vi "Signal Driver.vi"() -> ()   [LabVIEW 2010]
doc: "This version of Signal Driver uses a different file access option for method files and thus it can not open method files created with the previous version.\n\n\nSignal Driver is a general purpose signal generator that was designed to control experiments that required repeatable timing over widely varied time scales. Signal Driver provides an easy framework for creating analog waveforms that cycle on an off while retaining exact synchronization. Complex sequences of warm up and cycling of control signals during an experiment can be easily created using the warm up and program controls. The need for this software was Particle Tracking Velocimetry and Laser Induced Fluorescence in a wave tank. Signal Driver was designed to control the wavemaker, lasers, rotating mirror, shutter, and high speed digital camera while providing precise control of the phase relationships. \n\nThe main screen of the Signal Driver has 4 controls and a boolean control palette.\n\nramp time (s) - The number of seconds during which time the Analog output signals ramp to the last value in their waveform arrays. The ramping occurs using a sinusoidal curve. The ramping is designed to prevent damage to any devices that would suffer from a large instantaneous change in control voltage. Note that the ramp is to the LAST value, not to the first value in the waveform arrays. The assumption is that the waveforms are continuous and cyclic.\n\nWarm up - An array containg boolean switches for each of the channels as well as the number of times each element in the array is to be repeated.\n\nThe warm up control is the first part of the program and the array must contain at least one element. For each element in the warm up array Signal Driver writes one repeat period of signal to each channel n times based on the status of the boolean controls. Additional elements can be added by using the index control and then setting the boolean switches and n to the desired values. Channels that are turned off receive a constant analog voltage equal to the last voltage in their waveform array.\n\nRight click on the index to empty the array.\n\nProgram\nThe Program control is identical to the warm up control. The only difference is that the program cycles the number of times indicated by the program cycles control.\n\nProgram Cycles\nNumber of times that the program array is cycled through.\n\nControl Palette\nContains controls for setting waveforms, ramping to the start position, sending the programmed signals, ramping to zero, and quitting. The controls are dimmed when they are disabled."
uses:
  AO Write (waveform).vi
  AO Write (scaled array).vi
  wavecluster.ctl
  AO n wave.ctl
  SDMethod.ctl
panel:
  in  "Del warmup":bool
  in  "Del program":bool
  out "period (s)":dbl=2.0 format="%.2f"
  out "actual update rate":sgl=1000.0 format="%.8f"
  out "SD method":T1 {"method array"."offset" format="%.2f"; "method array"."amplitude" format="%.2f"; "method array"."cycles/repeat period" min=1}
  out "last value":dbl[](array[numeric])=[-6.999965667724609] format="%.2f"
  in  "program":T2[](array[typedef])=[{"n"=1, "on/off"=[TRUE, FALSE, FALSE, FALSE, FALSE, FALSE]}] {"n" min=1}
  out "ready to run":cluster{"ramped":bool, "got waveforms":bool}={"ramped"=FALSE, "got waveforms"=TRUE}
  out "delay":i32=500
  out "end of cycle":i32=1002
  out "program cycles done":i32(slide)=1 scale=0.0..1.0
  out "wave periods":i32=107
  in  "program cycles":i32=1 min=1
  in  "warm up":T2[](array[typedef])=[{"n"=1, "on/off"=[FALSE, FALSE, FALSE, FALSE, FALSE, FALSE]}] {"n" min=1}
  in  "buffer size":i32=2000
  in  "State":T3
  in  "ramp time (s)":dbl=2.0 min=1.0 step=0.1 format="%.1f"
  in  "ramp points":i32=1000 min=100 max=10000
  out "waveform array":T4=[[-7.0, -6.9999657, -6.9998617, -6.999689, -6.9994473, -6.9991364, -6.9987564, -6.998307, -6.9977894, -6.997202, -6.996546, -6.9958205, -6.995026, -6.994163, -6.9932303, -6.992229, -6.9911585, -6.9900193, -6.988811, -6.9875336, -6.986187, -6.9847717, -6.9832873, -6.9817343, -6.980112, -6.978421, -6.9766617, -6.974833, -6.972935, -6.9709687, -6.9689336, -6.96683, -6.9646573, -6.9624157, -6.9601054, -6.9577265, -6.9552794, -6.952763, -6.950178, -6.947525, -6.9448028, -6.9420123, -6.939153, -6.936226, -6.93323, -6.930166, -6.927033, -6.9238315, -6.9205623, -6.9172244, -6.9138184, -6.910344, -6.9068017, -6.903191, -6.8995123, -6.8957653, -6.89195, -6.8880672, -6.8841166, -6.8800974, -6.876011, -6.871856, -6.867634, -6.8633432, -6.8589854, -6.85456, -6.850066, -6.845505, -6.840877, -6.8361807, -6.8314176, -6.8265862, -6.821688, -6.8167224, -6.8116894, -6.8065896, -6.801422, -6.796188, -6.7908864, -6.7855177, -6.780082, -6.7745795, -6.7690105, -6.7633743, -6.7576714, -6.751902, -6.7460656, -6.740163, -6.734194, -6.728158, -6.722056, -6.715887, -6.7096524, -6.7033515, -6.6969843, -6.6905513, -6.684052, -6.6774864, -6.6708555, -6.6641583, -6.657396, -6.650567, -6.643673, -6.6367135, -6.6296883, -6.6225977, -6.6154413, -6.60822, -6.6009336, -6.593582, -6.5861654, -6.578684, -6.571137, -6.5635257, -6.555849, -6.548108, -6.5403028, -6.5324326, -6.524498, -6.5164986, -6.5084352, -6.500308, -6.492116, -6.4838605, -6.4755406, -6.467157, -6.4587092, -6.4501977, -6.4416227, -6.4329844, -6.4242826, -6.415517, -6.406688, -6.397796, -6.388841, -6.3798227, -6.370742, -6.361598, -6.352391, -6.3431215, -6.3337893, -6.3243947, -6.3149376, -6.3054185, -6.295837, -6.286193, -6.2764874, -6.2667193, -6.25689, -6.246999, -6.237046, -6.227031, -6.216955, -6.2068176, -6.196619, -6.1863594, -6.1760387, -6.1656566, -6.1552143, -6.144711, -6.1341467, -6.1235223, -6.1128373, -6.102092, -6.091286, -6.0804205, -6.0694947, -6.0585093, -6.047464, -6.036359, -6.025194, -6.01397, -6.0026865, -5.991344, -5.979942, -5.968481, -5.956961, -5.9453826, -5.9337454, -5.9220495, -5.9102955, -5.898483, -5.886612, -5.8746834, -5.862696, -5.8506517, -5.838549, -5.826389, -5.8141713, -5.801896, -5.789564, -5.7771745, -5.764728, -5.752225, -5.7396646, -5.727048, -5.7143745, -5.701645, -5.688859, -5.6760173, -5.663119, -5.650165, -5.637155, -5.6240897, -5.610969, -5.5977926, -5.584561, -5.5712743, -5.557933, -5.544536, -5.531085, -5.517579, -5.5040193, -5.4904046, -5.4767356, -5.4630127, -5.449236, -5.4354057, -5.421521, -5.4075837, -5.393593, -5.3795485, -5.365451, -5.3513007, -5.3370976, -5.3228416, -5.308533, -5.294173, -5.27976, -5.2652946, -5.2507777, -5.2362084, -5.221588, -5.206916, -5.1921926, -5.1774178, -5.162592, -5.147715, -5.132787, -5.1178093, -5.1027803, -5.0877013, -5.0725718, -5.0573926, -5.0421634, -5.026884, -5.011555, -4.996177, -4.9807496, -4.965273, -4.9497476, -4.934173, -4.91855, -4.9028783, -4.887158, -4.8713894, -4.855573, -4.839709, -4.8237967, -4.807837, -4.7918296, -4.7757754, -4.7596736, -4.743525, -4.7273297, -4.7110877, -4.694799, -4.678464, -4.662083, -4.645656, -4.6291833, -4.612664, -4.5961003, -4.5794907, -4.562836, -4.5461364, -4.529392, -4.5126023, -4.4957685, -4.4788904, -4.461968, -4.4450016, -4.427991, -4.4109373, -4.3938394, -4.3766985, -4.359514, -4.3422875, -4.3250175, -4.3077044, -4.2903495, -4.2729516, -4.255512, -4.2380304, -4.2205067, -4.2029414, -4.1853347, -4.167687, -4.1499977, -4.1322675, -4.1144967, -4.0966854, -4.0788336, -4.060941, -4.043009, -4.025037, -4.007025, -3.9889734, -3.9708827, -3.9527526, -3.9345837, -3.9163759, -3.8981292, -3.8798444, -3.861521, -3.8431597, -3.8247604, -3.8063233, -3.7878487, -3.7693367, -3.7507875, -3.7322013, -3.7135782, -3.6949186, -3.6762223, -3.65749, -3.6387215, -3.619917, -3.6010768, -3.582201, -3.5632899, -3.5443437, -3.5253625, -3.5063465, -3.4872956, -3.4682107, -3.4490914, -3.429938, -3.4107509, -3.39153, -3.3722758, -3.352988, -3.3336675, -3.314314, -3.2949276, -3.2755086, -3.2560575, -3.2365742, -3.2170591, -3.1975121, -3.1779335, -3.1583235, -3.1386826, -3.1190104, -3.0993075, -3.079574, -3.0598104, -3.0400164, -3.0201924, -3.0003386, -2.9804552, -2.9605422, -2.9406002, -2.920629, -2.900629, -2.8806005, -2.8605435, -2.8404584, -2.8203452, -2.800204, -2.7800353, -2.759839, -2.7396157, -2.7193651, -2.6990879, -2.6787841, -2.6584537, -2.638097, -2.6177144, -2.597306, -2.5768719, -2.5564122, -2.5359275, -2.5154178, -2.494883, -2.474324, -2.4537404, -2.4331324, -2.4125004, -2.3918447, -2.3711655, -2.3504627, -2.3297367, -2.3089879, -2.288216, -2.267422, -2.2466052, -2.2257664, -2.2049057, -2.1840231, -2.163119, -2.1421936, -2.1212468, -2.1002793, -2.079291, -2.0582824, -2.0372531, -2.0162039, -1.9951348, -1.974046, -1.9529377, -1.9318101, -1.9106636, -1.8894981, -1.8683139, -1.8471113, -1.8258905, -1.8046517, -1.783395, -1.7621208, -1.7408292, -1.7195204, -1.6981946, -1.6768521, -1.655493, -1.6341176, -1.612726, -1.5913185, -1.5698953, -1.5484567, -1.5270027, -1.5055337, -1.4840498, -1.4625512, -1.4410383, -1.4195111, -1.3979698, -1.3764149, -1.3548462, -1.3332644, -1.3116692, -1.2900611, -1.2684404, -1.246807, -1.2251614, -1.2035037, -1.1818341, -1.1601529, -1.1384602, -1.1167562, -1.0950413, -1.0733155, -1.0515791, -1.0298324, -1.0080755, -0.98630863, -0.964532, -0.9427459, -0.92095053, -0.899146, -0.8773326, -0.8555106, -0.8336801, -0.8118414, -0.7899947, -0.7681402, -0.7462781, -0.7244086, -0.702532, -0.68064845, -0.65875816, -0.63686144, -0.6149584, -0.5930492, -0.57113427, -0.54921365, -0.52728766, -0.50535643, -0.4834202, -0.4614792, -0.43953365, -0.41758376, -0.39562973, -0.37367183, -0.35171023, -0.32974514, -0.30777684, -0.28580546, -0.2638313, -0.24185449, -0.21987532, -0.19789396, -0.17591067, -0.15392563, -0.13193908, -0.10995122, -0.08796228, -0.06597247, -0.043982007, -0.021991113, 1.08586066e-13, 0.021991113, 0.043982007, 0.06597247, 0.08796228, 0.10995122, 0.13193908, 0.15392563, 0.17591067, 0.19789396, 0.21987532, 0.24185449, 0.2638313, 0.28580546, 0.30777684, 0.32974514, 0.35171023, 0.37367183, 0.39562973, 0.41758376, 0.43953365, 0.4614792, 0.4834202, 0.50535643, 0.52728766, 0.54921365, 0.57113427, 0.5930492, 0.6149584, 0.63686144, 0.65875816, 0.68064845, 0.702532, 0.7244086, 0.7462781, 0.7681402, 0.7899947, 0.8118414, 0.8336801, 0.8555106, 0.8773326, 0.899146, 0.92095053, 0.9427459, 0.964532, 0.98630863, 1.0080755, 1.0298324, 1.0515791, 1.0733155, 1.0950413, 1.1167562, 1.1384602, 1.1601529, 1.1818341, 1.2035037, 1.2251614, 1.246807, 1.2684404, 1.2900611, 1.3116692, 1.3332644, 1.3548462, 1.3764149, 1.3979698, 1.4195111, 1.4410383, 1.4625512, 1.4840498, 1.5055337, 1.5270027, 1.5484567, 1.5698953, 1.5913185, 1.612726, 1.6341176, 1.655493, 1.6768521, 1.6981946, 1.7195204, 1.7408292, 1.7621208, 1.783395, 1.8046517, 1.8258905, 1.8471113, 1.8683139, 1.8894981, 1.9106636, 1.9318101, 1.9529377, 1.974046, 1.9951348, 2.0162039, 2.0372531, 2.0582824, 2.079291, 2.1002793, 2.1212468, 2.1421936, 2.163119, 2.1840231, 2.2049057, 2.2257664, 2.2466052, 2.267422, 2.288216, 2.3089879, 2.3297367, 2.3504627, 2.3711655, 2.3918447, 2.4125004, 2.4331324, 2.4537404, 2.474324, 2.494883, 2.5154178, 2.5359275, 2.5564122, 2.5768719, 2.597306, 2.6177144, 2.638097, 2.6584537, 2.6787841, 2.6990879, 2.7193651, 2.7396157, 2.759839, 2.7800353, 2.800204, 2.8203452, 2.8404584, 2.8605435, 2.8806005, 2.900629, 2.920629, 2.9406002, 2.9605422, 2.9804552, 3.0003386, 3.0201924, 3.0400164, 3.0598104, 3.079574, 3.0993075, 3.1190104, 3.1386826, 3.1583235, 3.1779335, 3.1975121, 3.2170591, 3.2365742, 3.2560575, 3.2755086, 3.2949276, 3.314314, 3.3336675, 3.352988, 3.3722758, 3.39153, 3.4107509, 3.429938, 3.4490914, 3.4682107, 3.4872956, 3.5063465, 3.5253625, 3.5443437, 3.5632899, 3.582201, 3.6010768, 3.619917, 3.6387215, 3.65749, 3.6762223, 3.6949186, 3.7135782, 3.7322013, 3.7507875, 3.7693367, 3.7878487, 3.8063233, 3.8247604, 3.8431597, 3.861521, 3.8798444, 3.8981292, 3.9163759, 3.9345837, 3.9527526, 3.9708827, 3.9889734, 4.007025, 4.025037, 4.043009, 4.060941, 4.0788336, 4.0966854, 4.1144967, 4.1322675, 4.1499977, 4.167687, 4.1853347, 4.2029414, 4.2205067, 4.2380304, 4.255512, 4.2729516, 4.2903495, 4.3077044, 4.3250175, 4.3422875, 4.359514, 4.3766985, 4.3938394, 4.4109373, 4.427991, 4.4450016, 4.461968, 4.4788904, 4.4957685, 4.5126023, 4.529392, 4.5461364, 4.562836, 4.5794907, 4.5961003, 4.612664, 4.6291833, 4.645656, 4.662083, 4.678464, 4.694799, 4.7110877, 4.7273297, 4.743525, 4.7596736, 4.7757754, 4.7918296, 4.807837, 4.8237967, 4.839709, 4.855573, 4.8713894, 4.887158, 4.9028783, 4.91855, 4.934173, 4.9497476, 4.965273, 4.9807496, 4.996177, 5.011555, 5.026884, 5.0421634, 5.0573926, 5.0725718, 5.0877013, 5.1027803, 5.1178093, 5.132787, 5.147715, 5.162592, 5.1774178, 5.1921926, 5.206916, 5.221588, 5.2362084, 5.2507777, 5.2652946, 5.27976, 5.294173, 5.308533, 5.3228416, 5.3370976, 5.3513007, 5.365451, 5.3795485, 5.393593, 5.4075837, 5.421521, 5.4354057, 5.449236, 5.4630127, 5.4767356, 5.4904046, 5.5040193, 5.517579, 5.531085, 5.544536, 5.557933, 5.5712743, 5.584561, 5.5977926, 5.610969, 5.6240897, 5.637155, 5.650165, 5.663119, 5.6760173, 5.688859, 5.701645, 5.7143745, 5.727048, 5.7396646, 5.752225, 5.764728, 5.7771745, 5.789564, 5.801896, 5.8141713, 5.826389, 5.838549, 5.8506517, 5.862696, 5.8746834, 5.886612, 5.898483, 5.9102955, 5.9220495, 5.9337454, 5.9453826, 5.956961, 5.968481, 5.979942, 5.991344, 6.0026865, 6.01397, 6.025194, 6.036359, 6.047464, 6.0585093, 6.0694947, 6.0804205, 6.091286, 6.102092, 6.1128373, 6.1235223, 6.1341467, 6.144711, 6.1552143, 6.1656566, 6.1760387, 6.1863594, 6.196619, 6.2068176, 6.216955, 6.227031, 6.237046, 6.246999, 6.25689, 6.2667193, 6.2764874, 6.286193, 6.295837, 6.3054185, 6.3149376, 6.3243947, 6.3337893, 6.3431215, 6.352391, 6.361598, 6.370742, 6.3798227, 6.388841, 6.397796, 6.406688, 6.415517, 6.4242826, 6.4329844, 6.4416227, 6.4501977, 6.4587092, 6.467157, 6.4755406, 6.4838605, 6.492116, 6.500308, 6.5084352, 6.5164986, 6.524498, 6.5324326, 6.5403028, 6.548108, 6.555849, 6.5635257, 6.571137, 6.578684, 6.5861654, 6.593582, 6.6009336, 6.60822, 6.6154413, 6.6225977, 6.6296883, 6.6367135, 6.643673, 6.650567, 6.657396, 6.6641583, 6.6708555, 6.6774864, 6.684052, 6.6905513, 6.6969843, 6.7033515, 6.7096524, 6.715887, 6.722056, 6.728158, 6.734194, 6.740163, 6.7460656, 6.751902, 6.7576714, 6.7633743, 6.7690105, 6.7745795, 6.780082, 6.7855177, 6.7908864, 6.796188, 6.801422, 6.8065896, 6.8116894, 6.8167224, 6.821688, 6.8265862, 6.8314176, 6.8361807, 6.840877, 6.845505, 6.850066, 6.85456, 6.8589854, 6.8633432, 6.867634, 6.871856, 6.876011, 6.8800974, 6.8841166, 6.8880672, 6.89195, 6.8957653, 6.8995123, 6.903191, 6.9068017, 6.910344, 6.9138184, 6.9172244, 6.9205623, 6.9238315, 6.927033, 6.930166, 6.93323, 6.936226, 6.939153, 6.9420123, 6.9448028, 6.947525, 6.950178, 6.952763, 6.9552794, 6.9577265, 6.9601054, 6.9624157, 6.9646573, 6.96683, 6.9689336, 6.9709687, 6.972935, 6.974833, 6.9766617, 6.978421, 6.980112, 6.9817343, 6.9832873, 6.9847717, 6.986187, 6.9875336, 6.988811, 6.9900193, 6.9911585, 6.992229, 6.9932303, 6.994163, 6.995026, 6.9958205, 6.996546, 6.997202, 6.9977894, 6.998307, 6.9987564, 6.9991364, 6.9994473, 6.999689, 6.9998617, 6.9999657, 7.0, 6.9999657, 6.9998617, 6.999689, 6.9994473, 6.9991364, 6.9987564, 6.998307, 6.9977894, 6.997202, 6.996546, 6.9958205, 6.995026, 6.994163, 6.9932303, 6.992229, 6.9911585, 6.9900193, 6.988811, 6.9875336, 6.986187, 6.9847717, 6.9832873, 6.9817343, 6.980112, 6.978421, 6.9766617, 6.974833, 6.972935, 6.9709687, 6.9689336, 6.96683, 6.9646573, 6.9624157, 6.9601054, 6.9577265, 6.9552794, 6.952763, 6.950178, 6.947525, 6.9448028, 6.9420123, 6.939153, 6.936226, 6.93323, 6.930166, 6.927033, 6.9238315, 6.9205623, 6.9172244, 6.9138184, 6.910344, 6.9068017, 6.903191, 6.8995123, 6.8957653, 6.89195, 6.8880672, 6.8841166, 6.8800974, 6.876011, 6.871856, 6.867634, 6.8633432, 6.8589854, 6.85456, 6.850066, 6.845505, 6.840877, 6.8361807, 6.8314176, 6.8265862, 6.821688, 6.8167224, 6.8116894, 6.8065896, 6.801422, 6.796188, 6.7908864, 6.7855177, 6.780082, 6.7745795, 6.7690105, 6.7633743, 6.7576714, 6.751902, 6.7460656, 6.740163, 6.734194, 6.728158, 6.722056, 6.715887, 6.7096524, 6.7033515, 6.6969843, 6.6905513, 6.684052, 6.6774864, 6.6708555, 6.6641583, 6.657396, 6.650567, 6.643673, 6.6367135, 6.6296883, 6.6225977, 6.6154413, 6.60822, 6.6009336, 6.593582, 6.5861654, 6.578684, 6.571137, 6.5635257, 6.555849, 6.548108, 6.5403028, 6.5324326, 6.524498, 6.5164986, 6.5084352, 6.500308, 6.492116, 6.4838605, 6.4755406, 6.467157, 6.4587092, 6.4501977, 6.4416227, 6.4329844, 6.4242826, 6.415517, 6.406688, 6.397796, 6.388841, 6.3798227, 6.370742, 6.361598, 6.352391, 6.3431215, 6.3337893, 6.3243947, 6.3149376, 6.3054185, 6.295837, 6.286193, 6.2764874, 6.2667193, 6.25689, 6.246999, 6.237046, 6.227031, 6.216955, 6.2068176, 6.196619, 6.1863594, 6.1760387, 6.1656566, 6.1552143, 6.144711, 6.1341467, 6.1235223, 6.1128373, 6.102092, 6.091286, 6.0804205, 6.0694947, 6.0585093, 6.047464, 6.036359, 6.025194, 6.01397, 6.0026865, 5.991344, 5.979942, 5.968481, 5.956961, 5.9453826, 5.9337454, 5.9220495, 5.9102955, 5.898483, 5.886612, 5.8746834, 5.862696, 5.8506517, 5.838549, 5.826389, 5.8141713, 5.801896, 5.789564, 5.7771745, 5.764728, 5.752225, 5.7396646, 5.727048, 5.7143745, 5.701645, 5.688859, 5.6760173, 5.663119, 5.650165, 5.637155, 5.6240897, 5.610969, 5.5977926, 5.584561, 5.5712743, 5.557933, 5.544536, 5.531085, 5.517579, 5.5040193, 5.4904046, 5.4767356, 5.4630127, 5.449236, 5.4354057, 5.421521, 5.4075837, 5.393593, 5.3795485, 5.365451, 5.3513007, 5.3370976, 5.3228416, 5.308533, 5.294173, 5.27976, 5.2652946, 5.2507777, 5.2362084, 5.221588, 5.206916, 5.1921926, 5.1774178, 5.162592, 5.147715, 5.132787, 5.1178093, 5.1027803, 5.0877013, 5.0725718, 5.0573926, 5.0421634, 5.026884, 5.011555, 4.996177, 4.9807496, 4.965273, 4.9497476, 4.934173, 4.91855, 4.9028783, 4.887158, 4.8713894, 4.855573, 4.839709, 4.8237967, 4.807837, 4.7918296, 4.7757754, 4.7596736, 4.743525, 4.7273297, 4.7110877, 4.694799, 4.678464, 4.662083, 4.645656, 4.6291833, 4.612664, 4.5961003, 4.5794907, 4.562836, 4.5461364, 4.529392, 4.5126023, 4.4957685, 4.4788904, 4.461968, 4.4450016, 4.427991, 4.4109373, 4.3938394, 4.3766985, 4.359514, 4.3422875, 4.3250175, 4.3077044, 4.2903495, 4.2729516, 4.255512, 4.2380304, 4.2205067, 4.2029414, 4.1853347, 4.167687, 4.1499977, 4.1322675, 4.1144967, 4.0966854, 4.0788336, 4.060941, 4.043009, 4.025037, 4.007025, 3.9889734, 3.9708827, 3.9527526, 3.9345837, 3.9163759, 3.8981292, 3.8798444, 3.861521, 3.8431597, 3.8247604, 3.8063233, 3.7878487, 3.7693367, 3.7507875, 3.7322013, 3.7135782, 3.6949186, 3.6762223, 3.65749, 3.6387215, 3.619917, 3.6010768, 3.582201, 3.5632899, 3.5443437, 3.5253625, 3.5063465, 3.4872956, 3.4682107, 3.4490914, 3.429938, 3.4107509, 3.39153, 3.3722758, 3.352988, 3.3336675, 3.314314, 3.2949276, 3.2755086, 3.2560575, 3.2365742, 3.2170591, 3.1975121, 3.1779335, 3.1583235, 3.1386826, 3.1190104, 3.0993075, 3.079574, 3.0598104, 3.0400164, 3.0201924, 3.0003386, 2.9804552, 2.9605422, 2.9406002, 2.920629, 2.900629, 2.8806005, 2.8605435, 2.8404584, 2.8203452, 2.800204, 2.7800353, 2.759839, 2.7396157, 2.7193651, 2.6990879, 2.6787841, 2.6584537, 2.638097, 2.6177144, 2.597306, 2.5768719, 2.5564122, 2.5359275, 2.5154178, 2.494883, 2.474324, 2.4537404, 2.4331324, 2.4125004, 2.3918447, 2.3711655, 2.3504627, 2.3297367, 2.3089879, 2.288216, 2.267422, 2.2466052, 2.2257664, 2.2049057, 2.1840231, 2.163119, 2.1421936, 2.1212468, 2.1002793, 2.079291, 2.0582824, 2.0372531, 2.0162039, 1.9951348, 1.974046, 1.9529377, 1.9318101, 1.9106636, 1.8894981, 1.8683139, 1.8471113, 1.8258905, 1.8046517, 1.783395, 1.7621208, 1.7408292, 1.7195204, 1.6981946, 1.6768521, 1.655493, 1.6341176, 1.612726, 1.5913185, 1.5698953, 1.5484567, 1.5270027, 1.5055337, 1.4840498, 1.4625512, 1.4410383, 1.4195111, 1.3979698, 1.3764149, 1.3548462, 1.3332644, 1.3116692, 1.2900611, 1.2684404, 1.246807, 1.2251614, 1.2035037, 1.1818341, 1.1601529, 1.1384602, 1.1167562, 1.0950413, 1.0733155, 1.0515791, 1.0298324, 1.0080755, 0.98630863, 0.964532, 0.9427459, 0.92095053, 0.899146, 0.8773326, 0.8555106, 0.8336801, 0.8118414, 0.7899947, 0.7681402, 0.7462781, 0.7244086, 0.702532, 0.68064845, 0.65875816, 0.63686144, 0.6149584, 0.5930492, 0.57113427, 0.54921365, 0.52728766, 0.50535643, 0.4834202, 0.4614792, 0.43953365, 0.41758376, 0.39562973, 0.37367183, 0.35171023, 0.32974514, 0.30777684, 0.28580546, 0.2638313, 0.24185449, 0.21987532, 0.19789396, 0.17591067, 0.15392563, 0.13193908, 0.10995122, 0.08796228, 0.06597247, 0.043982007, 0.021991113, -6.395194e-13, -0.021991113, -0.043982007, -0.06597247, -0.08796228, -0.10995122, -0.13193908, -0.15392563, -0.17591067, -0.19789396, -0.21987532, -0.24185449, -0.2638313, -0.28580546, -0.30777684, -0.32974514, -0.35171023, -0.37367183, -0.39562973, -0.41758376, -0.43953365, -0.4614792, -0.4834202, -0.50535643, -0.52728766, -0.54921365, -0.57113427, -0.5930492, -0.6149584, -0.63686144, -0.65875816, -0.68064845, -0.702532, -0.7244086, -0.7462781, -0.7681402, -0.7899947, -0.8118414, -0.8336801, -0.8555106, -0.8773326, -0.899146, -0.92095053, -0.9427459, -0.964532, -0.98630863, -1.0080755, -1.0298324, -1.0515791, -1.0733155, -1.0950413, -1.1167562, -1.1384602, -1.1601529, -1.1818341, -1.2035037, -1.2251614, -1.246807, -1.2684404, -1.2900611, -1.3116692, -1.3332644, -1.3548462, -1.3764149, -1.3979698, -1.4195111, -1.4410383, -1.4625512, -1.4840498, -1.5055337, -1.5270027, -1.5484567, -1.5698953, -1.5913185, -1.612726, -1.6341176, -1.655493, -1.6768521, -1.6981946, -1.7195204, -1.7408292, -1.7621208, -1.783395, -1.8046517, -1.8258905, -1.8471113, -1.8683139, -1.8894981, -1.9106636, -1.9318101, -1.9529377, -1.974046, -1.9951348, -2.0162039, -2.0372531, -2.0582824, -2.079291, -2.1002793, -2.1212468, -2.1421936, -2.163119, -2.1840231, -2.2049057, -2.2257664, -2.2466052, -2.267422, -2.288216, -2.3089879, -2.3297367, -2.3504627, -2.3711655, -2.3918447, -2.4125004, -2.4331324, -2.4537404, -2.474324, -2.494883, -2.5154178, -2.5359275, -2.5564122, -2.5768719, -2.597306, -2.6177144, -2.638097, -2.6584537, -2.6787841, -2.6990879, -2.7193651, -2.7396157, -2.759839, -2.7800353, -2.800204, -2.8203452, -2.8404584, -2.8605435, -2.8806005, -2.900629, -2.920629, -2.9406002, -2.9605422, -2.9804552, -3.0003386, -3.0201924, -3.0400164, -3.0598104, -3.079574, -3.0993075, -3.1190104, -3.1386826, -3.1583235, -3.1779335, -3.1975121, -3.2170591, -3.2365742, -3.2560575, -3.2755086, -3.2949276, -3.314314, -3.3336675, -3.352988, -3.3722758, -3.39153, -3.4107509, -3.429938, -3.4490914, -3.4682107, -3.4872956, -3.5063465, -3.5253625, -3.5443437, -3.5632899, -3.582201, -3.6010768, -3.619917, -3.6387215, -3.65749, -3.6762223, -3.6949186, -3.7135782, -3.7322013, -3.7507875, -3.7693367, -3.7878487, -3.8063233, -3.8247604, -3.8431597, -3.861521, -3.8798444, -3.8981292, -3.9163759, -3.9345837, -3.9527526, -3.9708827, -3.9889734, -4.007025, -4.025037, -4.043009, -4.060941, -4.0788336, -4.0966854, -4.1144967, -4.1322675, -4.1499977, -4.167687, -4.1853347, -4.2029414, -4.2205067, -4.2380304, -4.255512, -4.2729516, -4.2903495, -4.3077044, -4.3250175, -4.3422875, -4.359514, -4.3766985, -4.3938394, -4.4109373, -4.427991, -4.4450016, -4.461968, -4.4788904, -4.4957685, -4.5126023, -4.529392, -4.5461364, -4.562836, -4.5794907, -4.5961003, -4.612664, -4.6291833, -4.645656, -4.662083, -4.678464, -4.694799, -4.7110877, -4.7273297, -4.743525, -4.7596736, -4.7757754, -4.7918296, -4.807837, -4.8237967, -4.839709, -4.855573, -4.8713894, -4.887158, -4.9028783, -4.91855, -4.934173, -4.9497476, -4.965273, -4.9807496, -4.996177, -5.011555, -5.026884, -5.0421634, -5.0573926, -5.0725718, -5.0877013, -5.1027803, -5.1178093, -5.132787, -5.147715, -5.162592, -5.1774178, -5.1921926, -5.206916, -5.221588, -5.2362084, -5.2507777, -5.2652946, -5.27976, -5.294173, -5.308533, -5.3228416, -5.3370976, -5.3513007, -5.365451, -5.3795485, -5.393593, -5.4075837, -5.421521, -5.4354057, -5.449236, -5.4630127, -5.4767356, -5.4904046, -5.5040193, -5.517579, -5.531085, -5.544536, -5.557933, -5.5712743, -5.584561, -5.5977926, -5.610969, -5.6240897, -5.637155, -5.650165, -5.663119, -5.6760173, -5.688859, -5.701645, -5.7143745, -5.727048, -5.7396646, -5.752225, -5.764728, -5.7771745, -5.789564, -5.801896, -5.8141713, -5.826389, -5.838549, -5.8506517, -5.862696, -5.8746834, -5.886612, -5.898483, -5.9102955, -5.9220495, -5.9337454, -5.9453826, -5.956961, -5.968481, -5.979942, -5.991344, -6.0026865, -6.01397, -6.025194, -6.036359, -6.047464, -6.0585093, -6.0694947, -6.0804205, -6.091286, -6.102092, -6.1128373, -6.1235223, -6.1341467, -6.144711, -6.1552143, -6.1656566, -6.1760387, -6.1863594, -6.196619, -6.2068176, -6.216955, -6.227031, -6.237046, -6.246999, -6.25689, -6.2667193, -6.2764874, -6.286193, -6.295837, -6.3054185, -6.3149376, -6.3243947, -6.3337893, -6.3431215, -6.352391, -6.361598, -6.370742, -6.3798227, -6.388841, -6.397796, -6.406688, -6.415517, -6.4242826, -6.4329844, -6.4416227, -6.4501977, -6.4587092, -6.467157, -6.4755406, -6.4838605, -6.492116, -6.500308, -6.5084352, -6.5164986, -6.524498, -6.5324326, -6.5403028, -6.548108, -6.555849, -6.5635257, -6.571137, -6.578684, -6.5861654, -6.593582, -6.6009336, -6.60822, -6.6154413, -6.6225977, -6.6296883, -6.6367135, -6.643673, -6.650567, -6.657396, -6.6641583, -6.6708555, -6.6774864, -6.684052, -6.6905513, -6.6969843, -6.7033515, -6.7096524, -6.715887, -6.722056, -6.728158, -6.734194, -6.740163, -6.7460656, -6.751902, -6.7576714, -6.7633743, -6.7690105, -6.7745795, -6.780082, -6.7855177, -6.7908864, -6.796188, -6.801422, -6.8065896, -6.8116894, -6.8167224, -6.821688, -6.8265862, -6.8314176, -6.8361807, -6.840877, -6.845505, -6.850066, -6.85456, -6.8589854, -6.8633432, -6.867634, -6.871856, -6.876011, -6.8800974, -6.8841166, -6.8880672, -6.89195, -6.8957653, -6.8995123, -6.903191, -6.9068017, -6.910344, -6.9138184, -6.9172244, -6.9205623, -6.9238315, -6.927033, -6.930166, -6.93323, -6.936226, -6.939153, -6.9420123, -6.9448028, -6.947525, -6.950178, -6.952763, -6.9552794, -6.9577265, -6.9601054, -6.9624157, -6.9646573, -6.96683, -6.9689336, -6.9709687, -6.972935, -6.974833, -6.9766617, -6.978421, -6.980112, -6.9817343, -6.9832873, -6.9847717, -6.986187, -6.9875336, -6.988811, -6.9900193, -6.9911585, -6.992229, -6.9932303, -6.994163, -6.995026, -6.9958205, -6.996546, -6.997202, -6.9977894, -6.998307, -6.9987564, -6.9991364, -6.9994473, -6.999689, -6.9998617, -6.9999657]] format="%.2f"
  in  "device (1)":i16=1
  in  "channels (0)":string[](array[string])=["0"]
  out "waveform graph":sgl[][](graph)=[[-6.9999657], [-6.9999485], [-6.9998965], [-6.99981], [-6.999689], [-6.9995337], [-6.999344], [-6.9991193], [-6.9988604], [-6.9985666], [-6.9982386], [-6.997876], [-6.997479], [-6.997047], [-6.996581], [-6.9960804], [-6.995545], [-6.994975], [-6.994371], [-6.9937325], [-6.993059], [-6.9923515], [-6.9916096], [-6.990833], [-6.9900217], [-6.9891763], [-6.9882965], [-6.987382], [-6.9864335], [-6.9854503], [-6.9844327], [-6.983381], [-6.982294], [-6.9811735], [-6.9800186], [-6.978829], [-6.9776053], [-6.9763474], [-6.9750547], [-6.973728], [-6.9723673], [-6.970972], [-6.9695425], [-6.9680786], [-6.966581], [-6.965049], [-6.9634824], [-6.9618816], [-6.960247], [-6.958578], [-6.956875], [-6.9551377], [-6.9533668], [-6.9515615], [-6.949722], [-6.947849], [-6.945941], [-6.944], [-6.942024], [-6.940015], [-6.937971], [-6.935894], [-6.9337826], [-6.931638], [-6.9294586], [-6.927246], [-6.924999], [-6.9227185], [-6.9204044], [-6.9180565], [-6.9156747], [-6.9132595], [-6.91081], [-6.9083276], [-6.905811], [-6.9032607], [-6.900677], [-6.89806], [-6.895409], [-6.892725], [-6.8900075], [-6.887256], [-6.8844714], [-6.8816533], [-6.878802], [-6.8759174], [-6.872999], [-6.8700476], [-6.867063], [-6.864045], [-6.8609943], [-6.85791], [-6.8547926], [-6.851642], [-6.848459], [-6.845242], [-6.8419924], [-6.83871], [-6.8353944], [-6.8320456], [-6.8286643], [-6.82525], [-6.821803], [-6.818323], [-6.8148108], [-6.8112655], [-6.8076873], [-6.8040767], [-6.8004336], [-6.7967577], [-6.7930493], [-6.7893085], [-6.7855353], [-6.7817297], [-6.777891], [-6.7740207], [-6.770118], [-6.766183], [-6.7622156], [-6.7582164], [-6.7541847], [-6.7501206], [-6.746025], [-6.741897], [-6.737737], [-6.7335453], [-6.7293215], [-6.725066], [-6.7207785], [-6.7164593], [-6.712108], [-6.7077255], [-6.7033114], [-6.6988654], [-6.694388], [-6.6898785], [-6.685338], [-6.680766], [-6.6761627], [-6.671528], [-6.666862], [-6.6621647], [-6.6574364], [-6.6526766], [-6.647886], [-6.643064], [-6.6382113], [-6.633327], [-6.6284122], [-6.623467], [-6.61849], [-6.613483], [-6.608445], [-6.6033764], [-6.598277], [-6.5931473], [-6.587987], [-6.582796], [-6.5775747], [-6.5723233], [-6.5670414], [-6.561729], [-6.5563865], [-6.551014], [-6.545611], [-6.5401783], [-6.534715], [-6.5292225], [-6.5236998], [-6.5181475], [-6.512565], [-6.5069532], [-6.5013113], [-6.4956403], [-6.489939], [-6.4842086], [-6.478449], [-6.4726596], [-6.466841], [-6.4609933], [-6.4551163], [-6.4492097], [-6.4432745], [-6.43731], [-6.4313164], [-6.4252944], [-6.419243], [-6.413163], [-6.4070544], [-6.4009166], [-6.3947506], [-6.388556], [-6.382333], [-6.376081], [-6.369801], [-6.363493], [-6.3571563], [-6.3507915], [-6.3443985], [-6.3379774], [-6.3315287], [-6.3250513], [-6.318547], [-6.312014], [-6.3054533], [-6.2988653], [-6.2922497], [-6.2856064], [-6.2789354], [-6.2722373], [-6.265512], [-6.258759], [-6.251979], [-6.2451715], [-6.238337], [-6.231476], [-6.2245874], [-6.2176723], [-6.21073], [-6.2037616], [-6.196766], [-6.189744], [-6.1826954], [-6.17562], [-6.1685185], [-6.161391], [-6.1542363], [-6.147056], [-6.1398497], [-6.132617], [-6.1253586], [-6.1180744], [-6.110764], [-6.103428], [-6.0960665], [-6.088679], [-6.081266], [-6.0738277], [-6.066364], [-6.058875], [-6.0513606], [-6.043821], [-6.0362563], [-6.0286665], [-6.021052], [-6.0134125], [-6.0057483], [-5.9980593], [-5.9903455], [-5.9826074], [-5.9748445], [-5.967057], [-5.9592457], [-5.95141], [-5.9435496], [-5.9356656], [-5.9277573], [-5.9198256], [-5.9118695], [-5.9038897], [-5.895886], [-5.887859], [-5.879808], [-5.8717337], [-5.863636], [-5.855515], [-5.8473706], [-5.8392034], [-5.8310127], [-5.822799], [-5.814563], [-5.806304], [-5.798022], [-5.789717], [-5.7813897], [-5.77304], [-5.7646675], [-5.756273], [-5.747856], [-5.739417], [-5.730956], [-5.7224727], [-5.7139673], [-5.7054405], [-5.696892], [-5.6883216], [-5.6797295], [-5.671116], [-5.662481], [-5.6538243], [-5.645147], [-5.6364484], [-5.6277285], [-5.6189876], [-5.6102257], [-5.6014433], [-5.59264], [-5.583816], [-5.5749717], [-5.5661063], [-5.557221], [-5.5483155], [-5.5393896], [-5.5304437], [-5.521477], [-5.512491], [-5.5034857], [-5.4944596], [-5.4854145], [-5.4763494], [-5.467265], [-5.4581614], [-5.449038], [-5.4398956], [-5.4307337], [-5.421553], [-5.4123535], [-5.4031353], [-5.393898], [-5.384642], [-5.3753676], [-5.3660746], [-5.356763], [-5.347433], [-5.338085], [-5.3287187], [-5.3193345], [-5.309932], [-5.3005123], [-5.2910748], [-5.281619], [-5.2721457], [-5.2626553], [-5.2531476], [-5.2436223], [-5.23408], [-5.22452], [-5.2149434], [-5.20535], [-5.1957397], [-5.1861124], [-5.176469], [-5.1668086], [-5.1571317], [-5.1474385], [-5.137729], [-5.1280036], [-5.118262], [-5.1085043], [-5.098731], [-5.0889416], [-5.079137], [-5.0693164], [-5.05948], [-5.049629], [-5.0397625], [-5.0298805], [-5.019984], [-5.0100718], [-5.0001445], [-4.990203], [-4.9802465], [-4.970276], [-4.96029], [-4.95029], [-4.940276], [-4.930248], [-4.920205], [-4.9101486], [-4.900078], [-4.8899937], [-4.8798957], [-4.869784], [-4.8596587], [-4.84952], [-4.8393683], [-4.829203], [-4.819025], [-4.8088336], [-4.7986293], [-4.7884126], [-4.7781825], [-4.7679405], [-4.7576857], [-4.7474184], [-4.7371387], [-4.726847], [-4.716543], [-4.7062273], [-4.6958995], [-4.6855597], [-4.6752086], [-4.6648455], [-4.654471], [-4.6440854], [-4.6336884], [-4.62328], [-4.6128607], [-4.6024303], [-4.591989], [-4.5815372], [-4.5710745], [-4.560601], [-4.5501175], [-4.5396233], [-4.529119], [-4.5186043], [-4.50808], [-4.4975452], [-4.487001], [-4.476447], [-4.4658833], [-4.45531], [-4.4447274], [-4.4341354], [-4.423534], [-4.412924], [-4.402304], [-4.391676], [-4.381039], [-4.3703933], [-4.359739], [-4.349076], [-4.3384047], [-4.3277254], [-4.3170376], [-4.3063416], [-4.295638], [-4.2849264], [-4.2742076], [-4.2634807], [-4.252746], [-4.242004], [-4.231255], [-4.2204986], [-4.209735], [-4.198964], [-4.188187], [-4.1774025], [-4.1666117], [-4.155814], [-4.1450105], [-4.1342], [-4.1233835], [-4.1125607], [-4.101732], [-4.090897], [-4.080056], [-4.06921], [-4.058358], [-4.0475006], [-4.036638], [-4.0257697], [-4.0148964], [-4.0040183], [-3.9931347], [-3.9822464], [-3.9713535], [-3.960456], [-3.9495537], [-3.938647], [-3.927736], [-3.9168208], [-3.9059014], [-3.8949783], [-3.884051], [-3.87312], [-3.8621855], [-3.851247], [-3.8403053], [-3.8293602], [-3.818412], [-3.8074605], [-3.796506], [-3.7855487], [-3.7745883], [-3.7636254], [-3.7526598], [-3.7416918], [-3.7307212], [-3.7197485], [-3.7087736], [-3.6977968], [-3.686818], [-3.675837], [-3.6648545], [-3.6538706], [-3.642885], [-3.631898], [-3.6209095], [-3.60992], [-3.5989294], [-3.5879378], [-3.5769453], [-3.565952], [-3.554958], [-3.5439637], [-3.532969], [-3.5219738], [-3.5109782], [-3.4999828], [-3.4889874], [-3.4779918], [-3.4669967], [-3.456002], [-3.4450076], [-3.4340136], [-3.4230204], [-3.4120278], [-3.4010363], [-3.3900456], [-3.3790562], [-3.3680677], [-3.3570807], [-3.346095], [-3.3351111], [-3.3241286], [-3.3131478], [-3.3021688], [-3.291192], [-3.2802172], [-3.2692444], [-3.2582738], [-3.2473059], [-3.2363403], [-3.2253773], [-3.214417], [-3.2034597], [-3.1925051], [-3.1815536], [-3.1706054], [-3.1596603], [-3.1487186], [-3.1377802], [-3.1268456], [-3.1159146], [-3.1049874], [-3.0940642], [-3.083145], [-3.0722296], [-3.0613186], [-3.050412], [-3.0395098], [-3.0286121], [-3.0177193], [-3.006831], [-2.9959476], [-2.9850693], [-2.974196], [-2.9633276], [-2.9524648], [-2.9416075], [-2.9307556], [-2.9199092], [-2.9090686], [-2.898234], [-2.8874052], [-2.8765824], [-2.8657658], [-2.8549554], [-2.8441515], [-2.833354], [-2.822563], [-2.8117788], [-2.8010013], [-2.7902308], [-2.7794673], [-2.7687109], [-2.7579615], [-2.7472198], [-2.7364852], [-2.7257583], [-2.715039], [-2.7043276], [-2.6936238], [-2.682928], [-2.6722405], [-2.661561], [-2.6508896], [-2.6402268], [-2.6295724], [-2.6189268], [-2.6082897], [-2.5976615], [-2.587042], [-2.5764318], [-2.5658305], [-2.5552385], [-2.5446558], [-2.5340824], [-2.5235188], [-2.5129647], [-2.5024204], [-2.491886], [-2.4813612], [-2.4708467], [-2.4603424], [-2.4498484], [-2.4393647], [-2.4288914], [-2.4184287], [-2.4079766], [-2.3975353], [-2.387105], [-2.3766856], [-2.3662775], [-2.3558803], [-2.3454945], [-2.3351202], [-2.3247573], [-2.314406], [-2.3040664], [-2.2937386], [-2.2834227], [-2.2731187], [-2.262827], [-2.2525473], [-2.24228], [-2.2320254], [-2.221783], [-2.2115533], [-2.2013361], [-2.191132], [-2.1809409], [-2.1707625], [-2.1605973], [-2.1504455], [-2.140307], [-2.1301818], [-2.12007], [-2.109972], [-2.0998876], [-2.0898173], [-2.0797606], [-2.0697181], [-2.0596898], [-2.0496755], [-2.0396755], [-2.02969], [-2.019719], [-2.0097625], [-1.999821], [-1.989894], [-1.9799821], [-1.9700851], [-1.9602033], [-1.9503366], [-1.9404852], [-1.9306493], [-1.9208288], [-1.9110239], [-1.9012346], [-1.8914613], [-1.8817036], [-1.8719621], [-1.8622365], [-1.8525271], [-1.842834], [-1.8331573], [-1.8234969], [-1.8138533], [-1.8042262], [-1.7946157], [-1.7850223], [-1.7754456], [-1.765886], [-1.7563435], [-1.7468182], [-1.7373103], [-1.7278197], [-1.7183466], [-1.7088912], [-1.6994534], [-1.6900332], [-1.680631], [-1.6712468], [-1.6618806], [-1.6525326], [-1.6432028], [-1.6338913], [-1.6245983], [-1.6153237], [-1.6060678], [-1.5968305], [-1.587612], [-1.5784124], [-1.5692317], [-1.5600702], [-1.5509278], [-1.5418046], [-1.5327007], [-1.5236162], [-1.5145513], [-1.5055059], [-1.4964802], [-1.4874743], [-1.4784883], [-1.4695222], [-1.4605762], [-1.4516503], [-1.4427445], [-1.4338591], [-1.4249941], [-1.4161496], [-1.4073256], [-1.3985224], [-1.3897398], [-1.3809781], [-1.3722372], [-1.3635174], [-1.3548187], [-1.3461411], [-1.3374848], [-1.3288498], [-1.3202363], [-1.3116443], [-1.3030739], [-1.2945251], [-1.2859981], [-1.277493], [-1.2690098], [-1.2605486], [-1.2521095], [-1.2436926], [-1.235298], [-1.2269258], [-1.218576], [-1.2102487], [-1.201944], [-1.1936619], [-1.1854026], [-1.1771662], [-1.1689527], [-1.1607622], [-1.1525948], [-1.1444505], [-1.1363297], [-1.1282319], [-1.1201577], [-1.1121069], [-1.1040797], [-1.0960761], [-1.0880964], [-1.0801404], [-1.0722082], [-1.0643], [-1.0564158], [-1.0485559], [-1.04072], [-1.0329084], [-1.0251212], [-1.0173584], [-1.0096202], [-1.0019065], [-0.99421746], [-0.98655313], [-0.9789136], [-0.971299], [-0.9637093], [-0.9561447], [-0.9486052], [-0.9410908], [-0.93360174], [-0.9261379], [-0.91869956], [-0.9112867], [-0.9038994], [-0.89653766], [-0.88920164], [-0.88189137], [-0.87460697], [-0.8673485], [-0.86011595], [-0.8529095], [-0.8457292], [-0.838575], [-0.8314471], [-0.8243456], [-0.81727046], [-0.8102218], [-0.8031997], [-0.7962042], [-0.7892354], [-0.7822934], [-0.77537817], [-0.7684898], [-0.76162845], [-0.75479406], [-0.7479868], [-0.7412067], [-0.73445386], [-0.7277283], [-0.72103006], [-0.7143593], [-0.707716], [-0.70110023], [-0.6945121], [-0.68795174], [-0.6814191], [-0.6749142], [-0.66843724], [-0.6619882], [-0.6555672], [-0.6491743], [-0.64280945], [-0.6364729], [-0.6301645], [-0.6238845], [-0.61763287], [-0.6114097], [-0.605215], [-0.5990489], [-0.5929114], [-0.58680266], [-0.58072263], [-0.5746714], [-0.56864905], [-0.5626556], [-0.5566912], [-0.55075586], [-0.5448496], [-0.5389725], [-0.5331246], [-0.527306], [-0.52151674], [-0.5157569], [-0.5100265], [-0.50432557], [-0.49865425], [-0.49301255], [-0.4874005], [-0.48181823], [-0.4762657], [-0.47074303], [-0.46525025], [-0.45978746], [-0.45435464], [-0.44895187], [-0.44357923], [-0.43823674], [-0.4329245], [-0.4276425], [-0.42239085], [-0.41716954], [-0.4119787], [-0.4068183], [-0.40168843], [-0.39658916], [-0.3915205], [-0.38648254], [-0.3814753], [-0.37649882], [-0.37155318], [-0.36663842], [-0.3617546], [-0.35690174], [-0.3520799], [-0.34728912], [-0.34252948], [-0.33780098], [-0.3331037], [-0.32843766], [-0.32380292], [-0.31919953], [-0.31462756], [-0.31008703], [-0.30557793], [-0.3011004], [-0.29665443], [-0.29224008], [-0.28785738], [-0.28350642], [-0.27918717], [-0.27489972], [-0.27064407], [-0.26642033], [-0.2622285], [-0.2580686], [-0.25394073], [-0.24984486], [-0.2457811], [-0.24174944], [-0.23774993], [-0.23378263], [-0.22984758], [-0.22594479], [-0.2220743], [-0.21823618], [-0.21443045], [-0.21065713], [-0.20691629], [-0.20320795], [-0.19953215], [-0.19588892], [-0.1922783], [-0.18870032], [-0.18515502], [-0.18164244], [-0.17816262], [-0.17471558], [-0.17130135], [-0.16791998], [-0.1645715], [-0.16125593], [-0.15797332], [-0.15472369], [-0.15150708], [-0.1483235], [-0.14517303], [-0.14205565], [-0.13897142], [-0.13592036], [-0.1329025], [-0.12991787], [-0.1269665], [-0.12404843], [-0.121163666], [-0.11831226], [-0.11549423], [-0.1127096], [-0.109958395], [-0.107240655], [-0.1045564], [-0.10190565], [-0.09928845], [-0.0967048], [-0.09415475], [-0.09163831], [-0.08915551], [-0.08670637], [-0.08429092], [-0.08190918], [-0.079561174], [-0.077246934], [-0.07496647], [-0.072719805], [-0.07050697], [-0.068327986], [-0.06618287], [-0.06407163], [-0.061994318], [-0.059950933], [-0.0579415], [-0.055966035], [-0.054024566], [-0.0521171], [-0.050243672], [-0.048404288], [-0.046598967], [-0.04482773], [-0.043090597], [-0.04138758], [-0.0397187], [-0.038083967], [-0.036483407], [-0.034917027], [-0.033384845], [-0.03188688], [-0.030423142], [-0.028993648], [-0.02759841], [-0.026237443], [-0.024910761], [-0.023618378], [-0.022360304], [-0.021136552], [-0.019947136], [-0.018792067], [-0.017671354], [-0.016585011], [-0.015533048], [-0.014515474], [-0.013532301], [-0.012583539], [-0.011669194], [-0.010789279], [-0.0099438], [-0.009132767], [-0.008356187], [-0.0076140678], [-0.0069064167], [-0.006233241], [-0.0055945474], [-0.0049903416], [-0.00442063], [-0.0038854186], [-0.003384712], [-0.0029185156], [-0.0024868336], [-0.0020896704], [-0.0017270303], [-0.0013989164], [-0.001105332], [-0.0008462803], [-0.00062176364], [-0.0004317842], [-0.00027634393], [-0.00015544436], [-6.9086665e-05], [-1.7271708e-05]]
  out "quit":bool=TRUE
  in  "Stop":bool
  # "Wave program status"
  # "The number of steps in the program are determined by the size of the program array!"
  # "hz"
  # "ticks"
  # "hz"
  # "ticks"
  # "ticks"
  # "volts"
  # "volts"
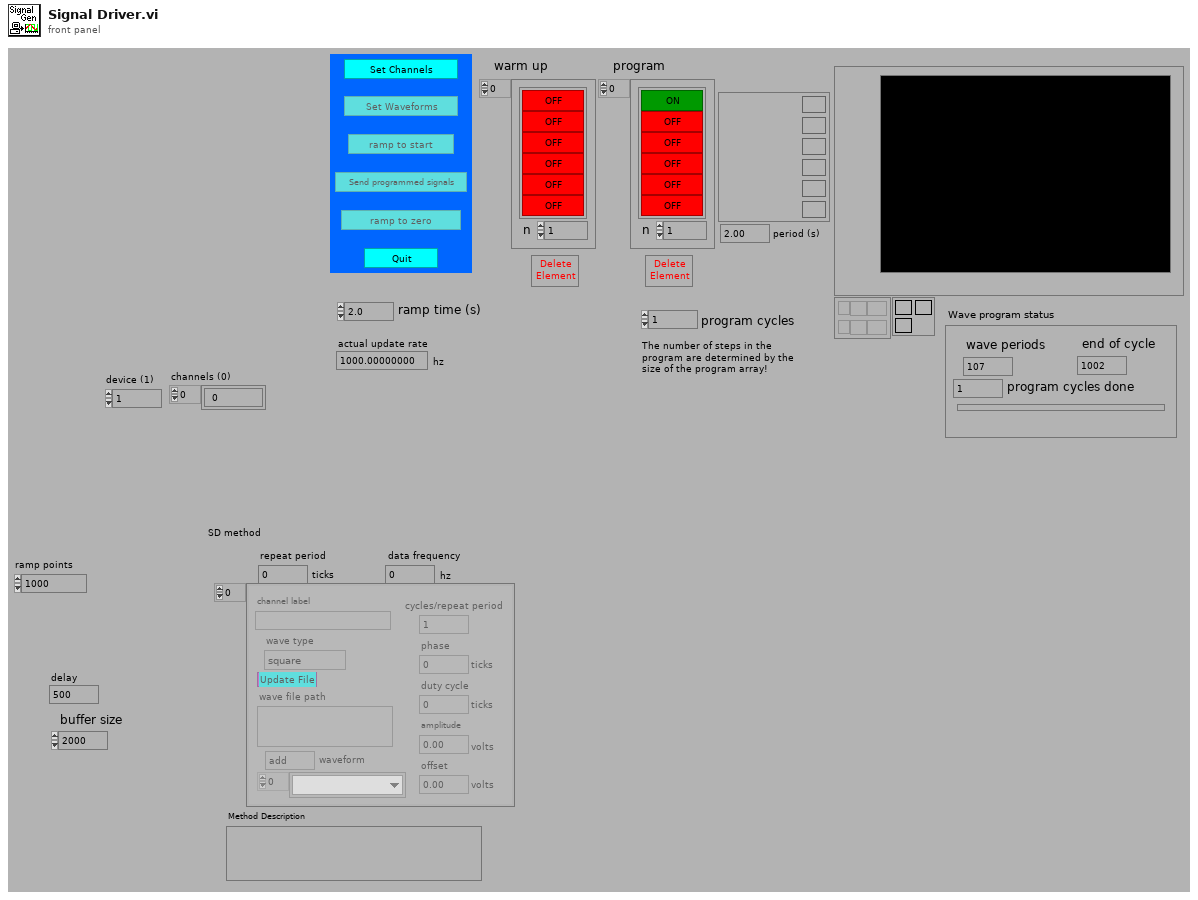
[diagram p1: front panel]
types:
  T1 = typedef "SDMethod.ctl" = cluster{"method array":cluster{"wave type":enum16{"off", "square", "sine", "triangle", "sawtooth", "from file", "wavemaker", "flume pump"}, "cycles/repeat period":u32, "phase":i32, "duty cycle":u32, "wave file path":path, "amplitude":dbl, "channel label":string, "Update":bool, "offset":dbl, " waveform":u16[], "Function":enum16{"add", "multiply"}}[], "Method Description":string, "data frequency":u32, "repeat period":u32}
  T2 = typedef "AO n wave.ctl" = cluster{"n":i32, "on/off":bool[]}
  T3 = cluster{"Quit":bool, "Set Channels":bool, "Set Waveforms":bool, "ramp up":bool, "send AO":bool, "ramp down":bool}
  T4 = typedef "wavecluster.ctl" = sgl[][]
  T5 = typedef "plot labels.ctl" = cluster{"name out":string[], "color out":u32[]}
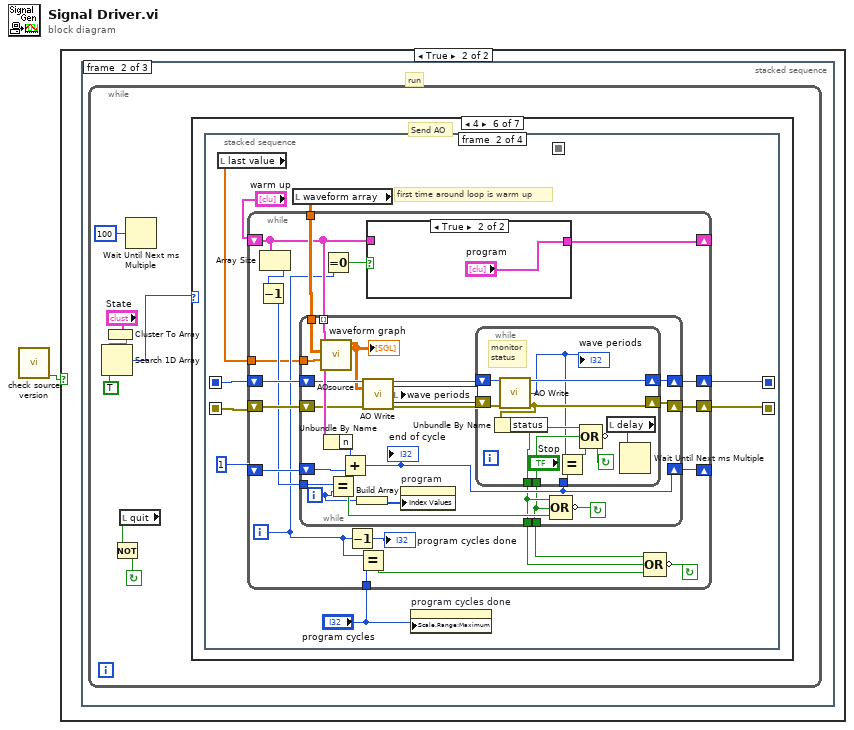
[diagram p0: block diagram]
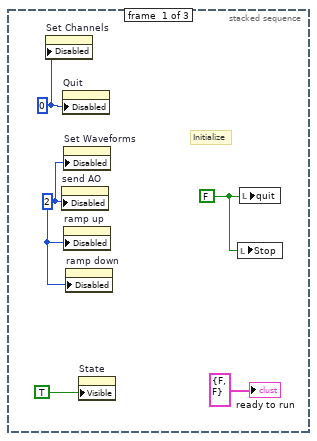
[diagram p3: hidden frame]
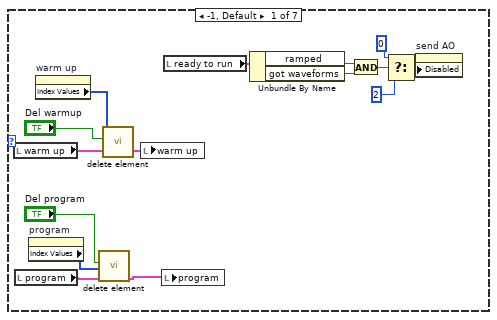
[diagram p4: hidden frame]
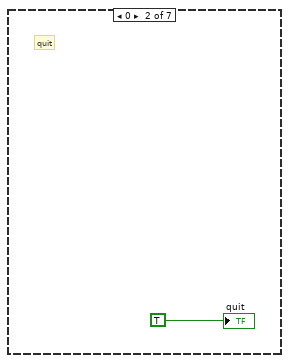
[diagram p5: hidden frame]
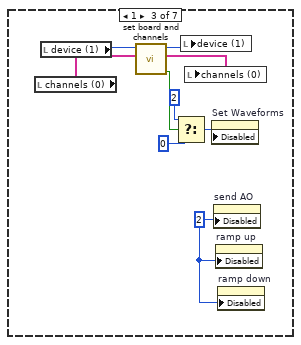
[diagram p6: hidden frame]
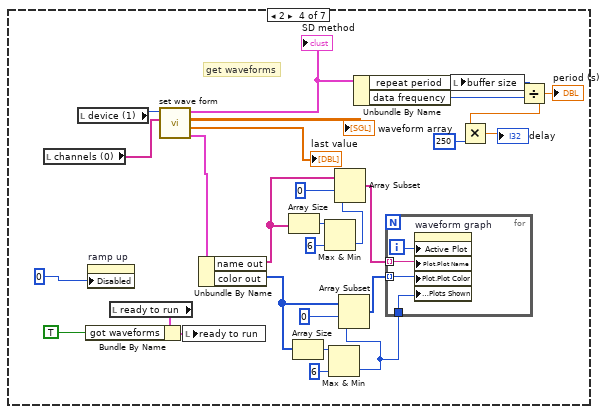
[diagram p7: hidden frame]
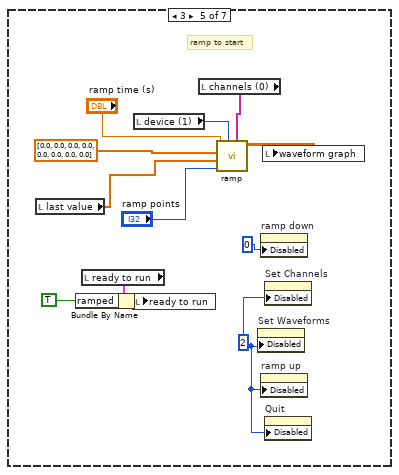
[diagram p8: hidden frame]
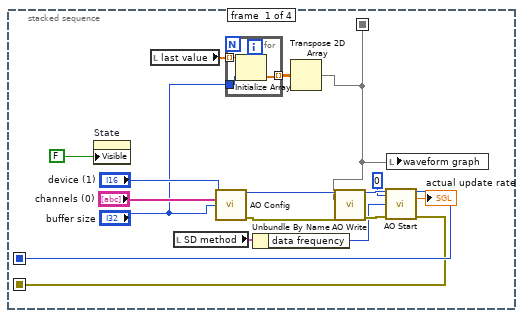
[diagram p9: hidden frame]
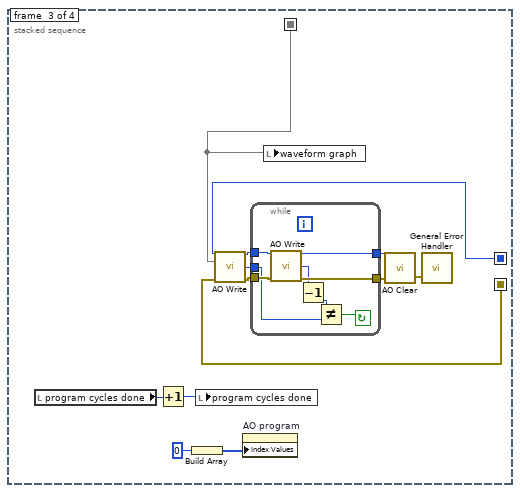
[diagram p11: hidden frame]
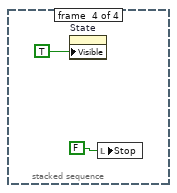
[diagram p12: hidden frame]
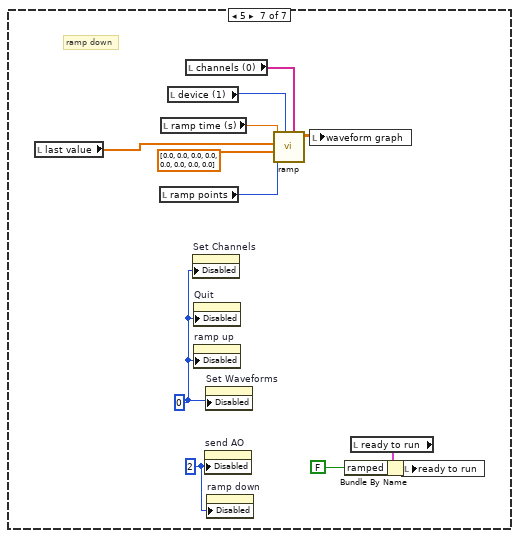
[diagram p13: hidden frame]
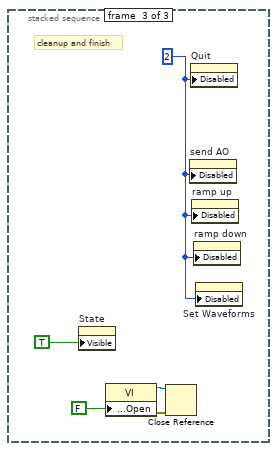
[diagram p14: hidden frame]
diagram:
  n1 = call "check source version.vi"() -> ("Accepted license"=w1:bool)  [unwired: 2 in, 3 out]
  n2 = case shown="True" w1 {
    frame False {
    }
    frame True {
      n3 = stacked-sequence {
        frame #0 {
          w2 = u8 0 ("Disabled")
          w3 = 2
          w5 = FALSE
          # "Initialize"
          n4 = property on="Set Channels" class="Bool"("Disabled"=w2) -> ()  [unwired: 2 in, 2 out]
          n5 = property on="send AO" class="Bool"("Disabled"=w3) -> ()  [unwired: 2 in, 2 out]
          n6 = property on="Quit" class="Bool"("Disabled"=w2) -> ()  [unwired: 2 in, 2 out]
          n7 = property on="Set Waveforms" class="Bool"("Disabled"=w3) -> ()  [unwired: 2 in, 2 out]
          n8 = property on="ramp up" class="Bool"("Disabled"=w3) -> ()  [unwired: 2 in, 2 out]
          n9 = property on="ramp down" class="Bool"("Disabled"=w3) -> ()  [unwired: 2 in, 2 out]
          n10 = property on="State" class="Clust"("Visible"=TRUE) -> ()  [unwired: 2 in, 2 out]
          n11 = local write "Stop"(w5) -> ()
          n12 = local write "quit"(w5) -> ()
          "ready to run" <- cluster{"ramped":bool, "set camera/laser":bool} {"ramped"=FALSE, "set camera/laser"=FALSE} ("ready to run")
        }
        frame #1 {
          # "run"
          n13 = while {
            stop <- w9 continue-if-true
            n14 = Cluster To Array(cluster="State") -> (array=w13:bool[])
            n15 = Search 1D Array(1D array=w13, element=TRUE) -> (index of element=w10:i32)  [unwired: 1 in]
            n16 = local read "quit"() -> (w8:bool)
            n17 = Not(x=w8) -> (.not. x?=w9:bool)
            n18 = Wait Until Next ms Multiple(millisecond multiple=u32 100) -> ()  [unwired: 1 out]
            n19 = case shown="4" w10 {
              frame -1, Default {
                n20 = local read "warm up"() -> (w18:T2[])
                n21 = local read "program"() -> (w19:T2[])
                n22 = property on="program" class="Arr (strict)"() -> ("Index Values"=w20:u32[])  [unwired: 2 in, 2 out]
                n23 = property on="warm up" class="Arr (strict)"() -> ("Index Values"=w16:u32[])  [unwired: 2 in, 2 out]
                n24 = call "delete element.vi"("program"=w19, "Del program"="Del program", "index value"=w20) -> ("program out"=w15:T2[])  [unwired: 8 in]
                n25 = call "delete element.vi"("program"=w18, "Del program"="Del warmup", "index value"=w16) -> ("program out"=w14:T2[])  [unwired: 8 in]
                n26 = local write "warm up"(w14) -> ()
                n27 = local write "program"(w15) -> ()
                n28 = local read "ready to run"() -> (w28:cluster{"ramped":bool, "got waveforms":bool})
                n29 = Unbundle By Name(w28) -> ("ramped"=w27:bool, "got waveforms"=w26:bool)
                n30 = And(x=w27, y=w26) -> (x .and. y?=w23:bool)
                n31 = Select(t=0, s=w23, f=2 ("t")) -> (s? t:f=w22:i32)
                n32 = property on="send AO" class="Bool"("Disabled"=w22) -> ()  [unwired: 2 in, 2 out]
              }
              frame 0 {
                # "quit"
                "quit" <- TRUE
              }
              frame 1 {
                w30 = 2
                n33 = local read "channels (0)"() -> (w35:string[])
                n34 = local read "device (1)"() -> (w36:i16)
                n35 = call "set board and channels.vi"("channels in"=w35, "device in"=w36) -> ("failed"=w34:bool, "channels out"=w38:string[], "device out"=w37:i16)  [unwired: 6 in, 1 out]
                n36 = Select(t=u8 2 ("Disabled"), s=w34, f=0) -> (s? t:f=w31:i32)
                n37 = local write "device (1)"(w37) -> ()
                n38 = local write "channels (0)"(w38) -> ()
                n39 = property on="Set Waveforms" class="Bool"("Disabled"=w31) -> ()  [unwired: 2 in, 2 out]
                n40 = property on="send AO" class="Bool"("Disabled"=w30) -> ()  [unwired: 2 in, 2 out]
                n41 = property on="ramp up" class="Bool"("Disabled"=w30) -> ()  [unwired: 2 in, 2 out]
                n42 = property on="ramp down" class="Bool"("Disabled"=w30) -> ()  [unwired: 2 in, 2 out]
              }
              frame 2 {
                # "get waveforms"
                n43 = local read "channels (0)"() -> (w52:string[])
                n44 = local read "device (1)"() -> (w53:i16)
                n45 = property on="ramp up" class="Bool"("Disabled"=0) -> ()  [unwired: 2 in, 2 out]
                n46 = local read "ready to run"() -> (w64:cluster{"ramped":bool, "got waveforms":bool})
                n47 = Bundle By Name(cluster=w64, "got waveforms"=TRUE ("ramped")) -> (w62:cluster{"ramped":bool, "got waveforms":bool})
                n48 = call "set wave form.vi"("channels (0)"=w52, "device (1)"=w53) -> ("plot labels"=w51:T5, "last value"=→"last value":dbl[], "waveforms"=→"waveform array":T4, "SD method out"=w60:T1)  [unwired: 6 in]
                "SD method" <- w60
                n49 = local write "ready to run"(w62) -> ()
                n50 = Unbundle By Name(w51) -> ("name out"=w40:string[], "color out"=w47:u32[])
                n51 = Array Size(array=w40) -> (size(s)=w44:i32)
                n52 = Array Size(array=w47) -> (size(s)=w49:i32)
                n53 = Max & Min(x=w44, y=6) -> (min(x,y)=w42:i32)  [unwired: 1 out]
                n54 = Max & Min(x=w49, y=6) -> (min(x,y)=w39:i32)  [unwired: 1 out]
                n55 = Array Subset(array=w40, index=0 ("Array Index"), length=w42) -> (w41:string[])
                n56 = Array Subset(array=w47, index=0 ("Array Index"), length=w39) -> (w46:u32[])
                n57 = Unbundle By Name(w60) -> ("repeat period"=w58:u32, "data frequency"=w57:u32)
                n58 = for {
                  tunnel: w41 -> [w68] mode=indexing
                  tunnel: w46 -> [w67] mode=indexing
                  tunnel: w39 -> [w66]
                  i -> [w69]
                  n59 = property on="waveform graph" class="WFGraph (strict)"("Active Plot"=w69, "Plot.Plot Name"=w68, "Plot.Plot Color"=w67, "Legend:Plots Shown"=w66) -> ()  [unwired: 2 in, 2 out]
                }
                n60 = local write "buffer size"(w58) -> ()
                n61 = Divide(x=w58, y=w57) -> (x/y=w56:dbl)
                "period (s)" <- w56
                n62 = Multiply(x=w56, y=250) -> (x*y=→"delay":dbl)
              }
              frame 3 {
                w70 = u8 2 ("Disabled")
                # "ramp to start"
                n63 = local read "last value"() -> (w72:dbl[])
                n64 = local read "ready to run"() -> (w75:cluster{"ramped":bool, "got waveforms":bool})
                n65 = Bundle By Name(cluster=w75, "ramped"=TRUE) -> (w73:cluster{"ramped":bool, "got waveforms":bool})
                n66 = local write "ready to run"(w73) -> ()
                n67 = local read "device (1)"() -> (w81:i16)
                n68 = local read "channels (0)"() -> (w71:string[])
                n69 = call "ramp.vi"("channels (0)"=w71, "device (1)"=w81, "points"="ramp points", "last value"=w72, "first value"=dbl[] [0.0, 0.0, 0.0, 0.0, 0.0, 0.0, 0.0, 0.0], "ramp time (s)"="ramp time (s)") -> ("ramp array"=w78:sgl[][])  [unwired: 4 in]
                n70 = property on="Set Waveforms" class="Bool"("Disabled"=w70) -> ()  [unwired: 2 in, 2 out]
                n71 = property on="ramp down" class="Bool"("Disabled"=u8 0) -> ()  [unwired: 2 in, 2 out]
                n72 = property on="ramp up" class="Bool"("Disabled"=w70) -> ()  [unwired: 2 in, 2 out]
                n73 = local write "waveform graph"(w78) -> ()
                n74 = property on="Set Channels" class="Bool"("Disabled"=w70) -> ()  [unwired: 2 in, 2 out]
                n75 = property on="Quit" class="Bool"("Disabled"=w70) -> ()  [unwired: 2 in, 2 out]
              }
              frame 4 {
                # "Send AO"
                n76 = stacked-sequence {
                  seq-local: [w90 _ _ _] -> [_ w108 _ _]
                  seq-local: [w89 _ _ _] -> [_ w110 _ _]
                  seq-local: [_ w104 _ _] -> [_ _ w176 _]
                  seq-local: [_ w105 _ _] -> [_ _ w177 _]
                  seq-local: [w83 _ _ _] -> [_ _ w168 _]
                  frame #0 {
                    n77 = property on="State" class="Clust"("Visible"=FALSE) -> ()  [unwired: 2 in, 2 out]
                    n78 = local read "last value"() -> (w86:dbl[])
                    n79 = local read "SD method"() -> (w88:T1)
                    n80 = call "AO Config.vi"("device (1)"="device (1)", "channels (0)"="channels (0)", "buffer size (1000 updates)"="buffer size") -> ("taskID"=w92:u32, "error out"=w91:errorcluster)  [unwired: 10 in, 1 out]
                    n81 = for {
                      tunnel: w86 -> [w101] mode=indexing
                      tunnel: "buffer size" -> [w100]
                      tunnel: [w99] -> w84 mode=indexing
                      n82 = Initialize Array(w101, w100) -> (w99:dbl[])
                    }
                    n83 = Unbundle By Name(w88) -> ("data frequency"=w87:u32)
                    n84 = Transpose 2D Array(2D array=w84) -> (transposed array=w83:dbl[][])
                    n85 = call-poly "AO Write.vi"("taskID in"=w92, "scaled data"=w83, "error in (no error)"=w91) -> ("taskID out"=w95:u32, "error out"=w94:errorcluster)  [unwired: 8 in, 3 out]
                    n86 = call "AO Start.vi"("taskID in"=w95, "number of buffer iterations (1)"=0, "update rate (1000 updates/sec)"=w87, "error in (no error)"=w94) -> ("taskID out"=w90:u32, "actual update rate"=→"actual update rate":sgl, "error out"=w89:errorcluster)  [unwired: 9 in]
                    n87 = local write "waveform graph"(w83) -> ()
                  }
                  frame #1 {
                    # "first time around loop is warm up"
                    n88 = local read "last value"() -> (w102:dbl[])
                    n89 = local read "waveform array"() -> (w109:T4)
                    n90 = while {
                      tunnel: w102 -> [w111]
                      shift-left: "warm up" -> [w116]
                      shift-right: [w117] -> _
                      tunnel: "program cycles" -> [w122]
                      shift-left: 1 -> [w125]
                      shift-right: [w124] -> _
                      shift-left: w108 -> [w126]
                      shift-right: [w127] -> w105
                      shift-left: w110 -> [w128]
                      shift-right: [w129] -> w104
                      tunnel: w109 -> [w130]
                      i -> [w112]
                      stop <- w123 continue-if-true
                      n91 = Array Size(array=w116) -> (size(s)=w115:i32)
                      n92 = Decrement(x=w115) -> (x-1=w114:i32)
                      n93 = while {
                        tunnel: w111 -> [w131]
                        tunnel: [w139] -> w119
                        tunnel: [w140] -> w120
                        shift-left: w125 -> [w143]
                        shift-right: [w141] -> w124
                        tunnel: w114 -> [w147]
                        tunnel: w130 -> [w132]
                        tunnel: w116 -> [w151] mode=indexing
                        shift-left: w128 -> [w144]
                        shift-right: [w150] -> w129
                        shift-left: w126 -> [w145]
                        shift-right: [w149] -> w127
                        i -> [w134]
                        stop <- w148 continue-if-true
                        n94 = call "AOsource.vi"("last value"=w131, "waveforms in"=w132, "AO"=w151) -> ("waveforms out"=w138:sgl[][])  [unwired: 8 in]
                        "waveform graph" <- w138
                        n95 = Unbundle By Name(w151) -> ("n"=w142:i32)
                        n96 = Equal?(x=w147, y=w134) -> (x = y?=w146:bool)
                        n97 = Add(x=w142, y=w143) -> (x+y=w141:i32)
                        "end of cycle" <- w141
                        n98 = Build Array(w134) -> (w133:i32[])
                        n99 = call-poly "AO Write.vi"("taskID in"=w145, "scaled data"=w138, "error in (no error)"=w144) -> ("taskID out"=w135:u32, "number of buffers done"=w136:i32, "error out"=w137:errorcluster)  [unwired: 8 in, 2 out]
                        n100 = local write "wave periods"(w136) -> ()
                        n101 = property on="program" class="Arr (strict)"("Index Values"=w133) -> ()  [unwired: 2 in, 2 out]
                        n102 = while {
                          tunnel: w141 -> [w155]
                          tunnel: ["Stop"] -> w139
                          tunnel: [w158] -> w140
                          shift-left: w137 -> [w161]
                          shift-right: [w159] -> w150
                          shift-left: w135 -> [w162]
                          shift-right: [w160] -> w149
                          stop <- w156 continue-if-true
                          # "monitor\nstatus"
                          n103 = call-poly "AO Write.vi"("taskID in"=w162, "error in (no error)"=w161) -> ("taskID out"=w160:u32, "number of buffers done"=w152:i32, "error out"=w159:errorcluster)  [unwired: 9 in, 2 out]
                          "wave periods" <- w152
                          n104 = Unbundle By Name(w159) -> ("status"=w158:bool)
                          n105 = Equal?(x=w152, y=w155) -> (x = y?=w157:bool)
                          n106 = Compound Arithmetic op=OR(w158, "Stop", w157) -> (invert w156:bool)
                          n107 = local read "delay"() -> (w153:i32)
                          n108 = Wait Until Next ms Multiple(millisecond multiple=w153) -> ()  [unwired: 1 out]
                        }
                        n109 = Compound Arithmetic op=OR(w140, w139, w146) -> (invert w148:bool)
                      }
                      n110 = Equal To 0?(x=w112) -> (x = 0?=w118:bool)
                      n111 = Decrement(x=w112) -> (x-1=→"program cycles done":i32)
                      n112 = Equal?(x=w112, y=w122) -> (x = y?=w121:bool)
                      n113 = case shown="True" w118 {
                        tunnel: w116 -> [w163 _]
                        tunnel: [w163 "program"] -> w117
                        frame False {
                        }
                        frame True {
                        }
                      }
                      n114 = Compound Arithmetic op=OR(w119, w120, w121) -> (invert w123:bool)
                    }
                    n115 = property on="program cycles done" class="Slide (strict)"("Scale.Range:Maximum"="program cycles") -> ()  [unwired: 2 in, 2 out]
                  }
                  frame #2 {
                    n116 = local read "program cycles done"() -> (w170:i32)
                    n117 = Increment(x=w170) -> (x+1=w166:i32)
                    n118 = Build Array(0) -> (w167:i32[])
                    n119 = local write "program cycles done"(w166) -> ()
                    n120 = call-poly "AO Write.vi"("taskID in"=w177, "scaled data"=w168, "error in (no error)"=w176) -> ("taskID out"=w174:u32, "number of buffers done"=w169:i32, "error out"=w172:errorcluster)  [unwired: 8 in, 2 out]
                    n121 = property on="AO program" class="Arr (strict)"("Index Values"=w167) -> ()  [unwired: 2 in, 2 out]
                    n122 = while {
                      tunnel: w169 -> [w179]
                      tunnel: [w182] -> w171
                      tunnel: w172 -> [w183]
                      tunnel: [w184] -> w173
                      tunnel: w174 -> [w185]
                      stop <- w178 continue-if-true
                      n123 = call-poly "AO Write.vi"("taskID in"=w185, "error in (no error)"=w183) -> ("taskID out"=w184:u32, "number of buffers done"=w180:i32, "error out"=w182:errorcluster)  [unwired: 9 in, 2 out]
                      n124 = Decrement(x=w180) -> (x-1=w181:i32)
                      n125 = Not Equal?(x=w181, y=w179) -> (x != y?=w178:bool)
                    }
                    n126 = local write "waveform graph"(w168) -> ()
                    n127 = call "AO Clear.vi"("error in (no error)"=w171, "taskID in"=w173) -> ("error out"=w175:errorcluster)  [unwired: 4 in, 1 out]
                    n128 = call <vilib>:"General Error Handler.vi"("error in (no error)"=w175) -> ()  [unwired: 10 in, 5 out]
                  }
                  frame #3 {
                    n129 = property on="State" class="Clust"("Visible"=TRUE) -> ()  [unwired: 2 in, 2 out]
                    n130 = local write "Stop"(FALSE) -> ()
                  }
                }
              }
              frame 5 {
                w194 = u8 2 ("Disabled")
                w188 = u8 0 ("Disabled")
                # "ramp down"
                n131 = local read "last value"() -> (w190:dbl[])
                n132 = local read "ramp points"() -> (w195:i32)
                n133 = local read "ramp time (s)"() -> (w198:dbl)
                n134 = local read "device (1)"() -> (w197:i16)
                n135 = local read "channels (0)"() -> (w196:string[])
                n136 = property on="Set Channels" class="Bool"("Disabled"=w188) -> ()  [unwired: 2 in, 2 out]
                n137 = property on="Quit" class="Bool"("Disabled"=w188) -> ()  [unwired: 2 in, 2 out]
                n138 = property on="ramp up" class="Bool"("Disabled"=w188) -> ()  [unwired: 2 in, 2 out]
                n139 = property on="send AO" class="Bool"("Disabled"=w194) -> ()  [unwired: 2 in, 2 out]
                n140 = property on="Set Waveforms" class="Bool"("Disabled"=w188) -> ()  [unwired: 2 in, 2 out]
                n141 = property on="ramp down" class="Bool"("Disabled"=w194) -> ()  [unwired: 2 in, 2 out]
                n142 = call "ramp.vi"("channels (0)"=w196, "device (1)"=w197, "points"=w195, "last value"=dbl[] [0.0, 0.0, 0.0, 0.0, 0.0, 0.0, 0.0, 0.0] ("first value"), "first value"=w190, "ramp time (s)"=w198) -> ("ramp array"=w199:sgl[][])  [unwired: 4 in]
                n143 = local write "waveform graph"(w199) -> ()
                n144 = local read "ready to run"() -> (w193:cluster{"ramped":bool, "got waveforms":bool})
                n145 = Bundle By Name(cluster=w193, "ramped"=FALSE) -> (w191:cluster{"ramped":bool, "got waveforms":bool})
                n146 = local write "ready to run"(w191) -> ()
              }
            }
          }
        }
        frame #2 {
          w203 = 2
          # "cleanup and finish"
          n147 = property on="State" class="Clust"("Visible"=TRUE) -> ()  [unwired: 2 in, 2 out]
          n148 = property class="VI"("Front Panel Window:Open"=FALSE) -> (reference out=w200:refnum<vi>, error out=w201:errorcluster)  [unwired: 2 in]
          n149 = Close Reference(reference=w200, error in (no error)=w201) -> ()  [unwired: 1 out]
          n150 = property on="send AO" class="Bool"("Disabled"=w203) -> ()  [unwired: 2 in, 2 out]
          n151 = property on="Quit" class="Bool"("Disabled"=w203) -> ()  [unwired: 2 in, 2 out]
          n152 = property on="ramp up" class="Bool"("Disabled"=w203) -> ()  [unwired: 2 in, 2 out]
          n153 = property on="ramp down" class="Bool"("Disabled"=w203) -> ()  [unwired: 2 in, 2 out]
          n154 = property on="Set Waveforms" class="Bool"("Disabled"=w203) -> ()  [unwired: 2 in, 2 out]
        }
      }
    }
  }
